vi "UpdateFPGA.vi"(8 "error in (no error)":errorcluster, 10 "FPGA ScanControl In":T2, 11 "Refnum in":refnum<k20>) -> (0 "error out":errorcluster, 2 "FPGA Timing out":T1={"Sweep frequency (kHz)"=625.0, "Fast scanner frequency (kHz)"=2.0833333333333335, "Volume frequency (Hz)"=27.778317911737172} {"Volume frequency (Hz)" format="%_6g"; "Fast scanner frequency (kHz)" format="%_6g"; "Sweep frequency (kHz)" format="%_6g"}, 3 "Refnum out":refnum<k20>)   [LabVIEW 2016]
uses:
  CTL/FPGA_ScanControl.ctl
  CTL/FPGA_Timing.ctl
  <vilib>/Utility/error.llb/Error Cluster From Error Code.vi
  <vilib>/rvi/errors/niLvFpgaAdjustHostInterfaceError.vi
  <vilib>/rvi/interface/nirviReadWriteControl/nirviReadWriteControl.xnode
  NiFpgaLv.dll
  <vilib>/rvi/interface/Simulation/niFpgaSimulationCallBeginRW.vi
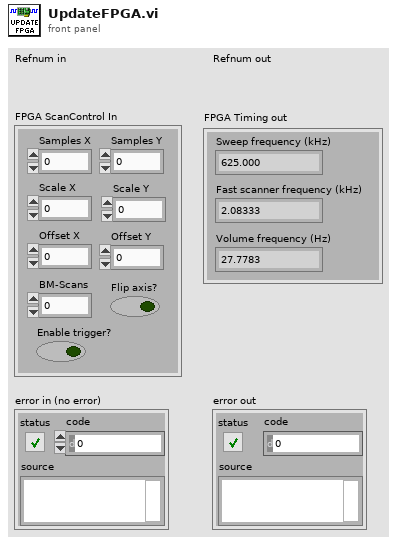
[diagram p1: front panel]
types:
  T1 = typedef "FPGA_Timing.ctl" = cluster{"Sweep frequency (kHz)":dbl, "Fast scanner frequency (kHz)":dbl, "Volume frequency (Hz)":dbl}
  T2 = typedef "FPGA_ScanControl.ctl" = cluster{"Samples X":i16, "Scale X":i16, "Offset X":i16, "Samples Y":i16, "Scale Y":i16, "Offset Y":i16, "BM-Scans":i16, "Flip axis?":bool, "Enable trigger?":bool}
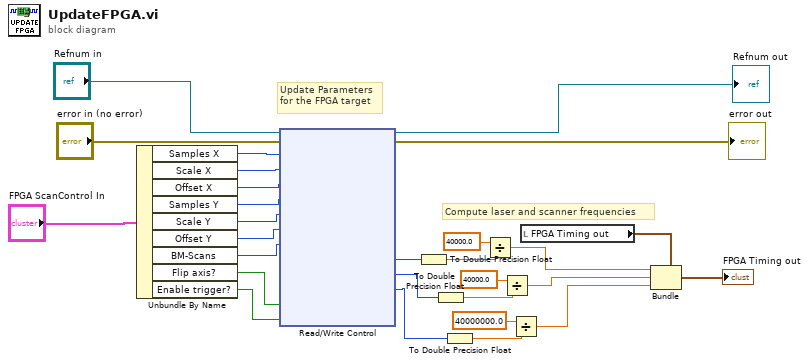
[diagram p0: block diagram]
diagram:
  # "Compute laser and scanner frequencies"
  # "Update Parameters\nfor the FPGA target"
  n1 = Unbundle By Name("FPGA ScanControl In") -> ("Samples X"=w20:i16, "Scale X"=w21:i16, "Offset X"=w22:i16, "Samples Y"=w23:i16, "Scale Y"=w24:i16, "Offset Y"=w25:i16, "BM-Scans"=w26:i16, "Flip axis?"=w27:bool, "Enable trigger?"=w28:bool)
  n2 = xnode "Read/Write Control"("FPGA VI Reference In"="Refnum in", "error in"="error in (no error)", "Samples X"=w20, "Scale X"=w21, "Offset X"=w22, "Samples Y"=w23, "Scale Y"=w24, "Offset Y"=w25, "BM-Scans"=w26, "Flip axis?"=w27, "Enable trigger?"=w28) -> ("FPGA VI Reference Out"=→"Refnum out":refnum<k20>, "error out"=→"error out":errorcluster, "Laser clock (ticks)"=w8:u32, "Fast period (ticks)"=w12:u32, "Slow period (ticks)"=w15:u32)
  n3 = To Double Precision Float(number=w8) -> (double precision float=w9:dbl)
  n4 = To Double Precision Float(number=w12) -> (double precision float=w11:dbl)
  n5 = To Double Precision Float(number=w15) -> (double precision float=w14:dbl)
  n6 = Divide(x=40000.0, y=w9) -> (x/y=w16:dbl)
  n7 = Divide(x=40000.0, y=w11) -> (x/y=w17:dbl)
  n8 = Divide(x=40000000.0, y=w14) -> (x/y=w18:dbl)
  n9 = local read "FPGA Timing out"() -> (w1:T1)
  n10 = Bundle(cluster=w1, "Sweep frequency (kHz)"=w16, "Fast scanner frequency (kHz)"=w17, "Volume frequency (Hz)"=w18) -> (→"FPGA Timing out":T1)
